vi "Standalone Destroy.vi"(6 "Standalone?":bool, 8 "error in (no error)":errorcluster, 9 "Event-Registrations In":T1, 11 "Actor in":refnum<class "Actor.lvclass">) -> (0 "error out":errorcluster, 3 "Actor out":refnum<class "Actor.lvclass">)   [LabVIEW 2018, in "Actor.lvclass"]
uses:
  Actor.lvclass
  Event-Registrations.ctl
  Stop.ctl
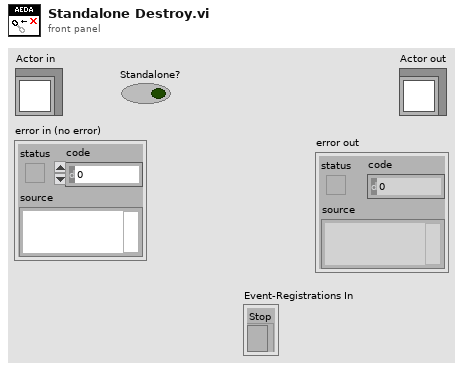
[diagram p1: front panel]
types:
  T1 = typedef "Actor.lvclass/Event-Registrations.ctl" = cluster{"Stop":refnum<event-registration>}
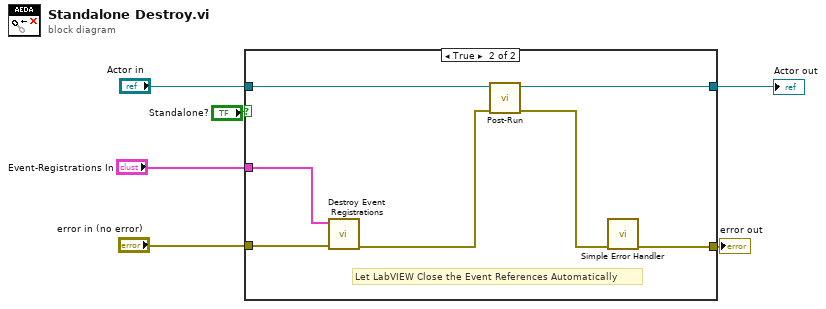
[diagram p0: block diagram]
diagram:
  n1 = case shown="True" "Standalone?" {
    tunnel: "Actor in" -> [w8 w13]
    tunnel: "error in (no error)" -> [w7 w15]
    tunnel: [w7 w9] -> w4
    tunnel: [w8 w11] -> w3
    tunnel: "Event-Registrations In" -> [_ w14]
    frame False {
    }
    frame True {
      # "Let LabVIEW Close the Event References Automatically"
      n2 = call "Destroy Event Registrations.vi"("error in (no error)"=w15, "Event-Registrations"=w14) -> ("error out"=w10:errorcluster)  [unwired: 9 in]
      n3 = call-dynamic "Post-Run.vi"("error in"=w10, "Actor in"=w13) -> ("error out"=w12:errorcluster, "Actor out"=w11:refnum<class "Actor.lvclass">)  [unwired: 8 in]
      n4 = call <vilib>:"Simple Error Handler.vi"("error in (no error)"=w12) -> ("error out"=w9:errorcluster)  [unwired: 4 in, 4 out]
    }
  }
  "error out" <- w4
  "Actor out" <- w3
